vi "Close Progress Bar.vi"(8 "error in (no error)":errorcluster, 11 "Progress Bar Dialog":refnum<class "Progress Bar Dialog.lvclass">) -> (0 "error out":errorcluster)   [LabVIEW 2020, in "Progress Bar Dialog.lvclass"]
doc: "This VI increments the progress bar one final time and closes the references associated with the progress bar."
uses:
  <vilib>/ProgressBar/Progress Bar Dialog.lvclass
  <vilib>/ProgressBar/Progress Bar Dialog.lvclass/Progress Bar Dialog.ctl
panel:
  in  "Load Complete":string="Load Complete"
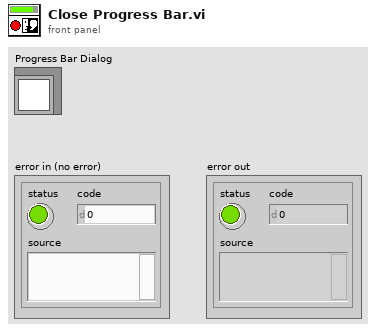
[diagram p1: front panel]
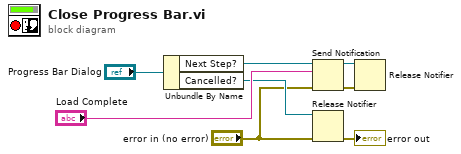
[diagram p0: block diagram]
diagram:
  n1 = Unbundle By Name("Progress Bar Dialog") -> ("Next Step?"=w4:refnum<notifier>, "Cancelled?"=w3:refnum<notifier>)
  n2 = Send Notification(notification="Load Complete", notifier=w4, error in (no error)="error in (no error)") -> (notifier out=w6:refnum<notifier>, error out=w8:errorcluster)
  n3 = Release Notifier(notifier=w3, error in (no error)="error in (no error)") -> (error out=→"error out":errorcluster)  [unwired: 1 in, 2 out]
  n4 = Release Notifier(notifier=w6, error in (no error)=w8) -> ()  [unwired: 1 in, 3 out]
